vi "Sort SR List.vi"(8 "Sorting":T1, 11 "list in":T2[](array[typedef]) {"Creation Date" format="%<%x>T"; "Last Updated" format="%<%x>T"}) -> (3 "list out":T2[](array[typedef]) {"Creation Date" format="%<%x>T"; "Last Updated" format="%<%x>T"})   [LabVIEW 2018]
uses:
  Type Defs/SR Cluster.ctl
  Type Defs/SR Status.ctl
  Type Defs/Sorting Methods.ctl
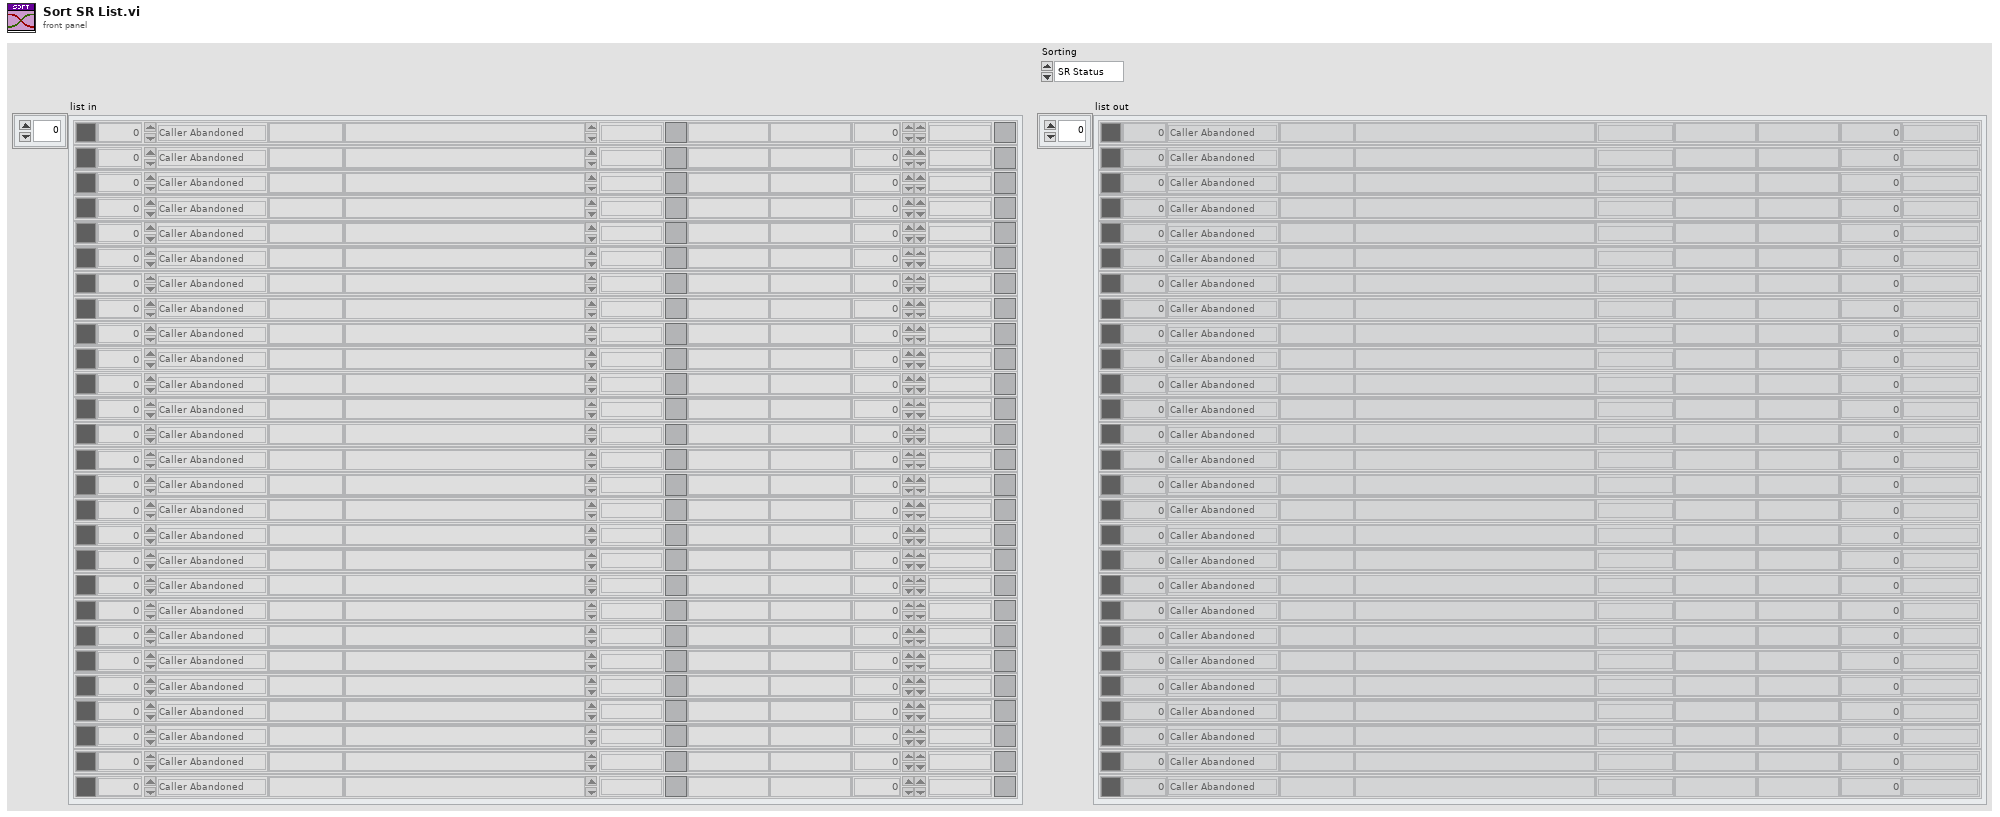
[diagram p1: front panel]
types:
  T1 = typedef "Sorting Methods.ctl" = enum16{"SR Status", "Most Recent", "SR Type", "SR Number", "Days Open", "Urgency"}
  T2 = typedef "SR Cluster.ctl" = cluster{"Color":u32, "SR Number":i32, "SR Status":T3, "Name":string, "Summary":string, "Last Updated":timestamp, "SR Type":string, "Service Level":string, "Days Open":dbl, "Creation Date":timestamp}
  T3 = typedef "SR Status.ctl" = enum16{"Caller Abandoned", "Created in Error", "Expired", "Forum Resolved AE", "Forum Resolved Customer", "IN WORK", "IN WORK Collab with AES", "IN WORK Collab with PSE", "IN WORK Collab with SE", "IN WORK Customer Added Note", "IN WORK Escalation", "IN WORK Wait on Customer", "Open", "Potentially Resolved", "Presumed Resolved", "RMA Approved for Return", "RMA Closed", "RMA Closed - DOA", "RMA In Progress", "RMA Open", "RMA Waiting on Customer", "Resolved", "Passed Off"}
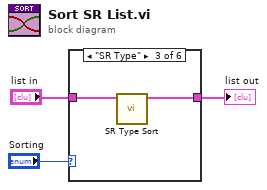
[diagram p0: block diagram]
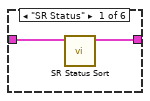
[diagram p2: hidden frame]
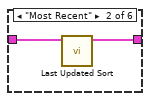
[diagram p3: hidden frame]
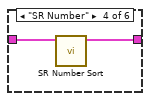
[diagram p4: hidden frame]
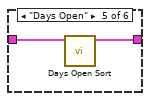
[diagram p5: hidden frame]
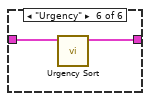
[diagram p6: hidden frame]
diagram:
  n1 = case shown="\"SR Type\"" "Sorting" {
    tunnel: "list in" -> [w5 w7 w9 w11 w13 w15]
    tunnel: [w4 w6 w8 w10 w12 w14] -> w1
    frame "SR Status" {
      n2 = call "SR Status Sort.vi"("list in"=w5) -> ("Array"=w4:T2[])  [unwired: 10 in]
    }
    frame "Most Recent" {
      n3 = call "Last Updated Sort.vi"("list in"=w7) -> ("Array"=w6:T2[])  [unwired: 10 in]
    }
    frame "SR Type" {
      n4 = call "SR Type Sort.vi"("list in"=w9) -> ("Array"=w8:T2[])  [unwired: 10 in]
    }
    frame "SR Number" {
      n5 = call "SR Number Sort.vi"("list in"=w11) -> ("Array"=w10:T2[])  [unwired: 10 in]
    }
    frame "Days Open" {
      n6 = call "Days Open Sort.vi"("list in"=w13) -> ("Array"=w12:T2[])  [unwired: 10 in]
    }
    frame "Urgency" {
      n7 = call "Urgency Sort.vi"("list in"=w15) -> ("Array"=w14:T2[])  [unwired: 10 in]
    }
  }
  "list out" <- w1
